vi "PIDAutoTune_OpenLoopStep.vi"(7 "Configuration Parameters":T2={"Controller Constant Type"=enum."Ziegler Nicols - Normal", "Type of Controller"=enum."PI", "CO Offset"=0.25, "Kn"=1.0, "Tuning Tolerance"=0.001, "Plant Tolerance"=0.001, "Newest Avg Time "=1, "Long Ave Time"=6}, 8 "Sampling Time dt (s)":dbl=0.02, 9 "Tune":bool, 10 "Measurement  (PV)":dbl, 11 "Control Output (Co)":dbl) -> (0 "Plant and Test Data":T4, 1 "New Tuning Parameters":T3, 2 "Tuning Done":bool, 3 "Adj CO":dbl, 4 "Error Occured":bool, 6 "Diagnostic":T1)   [LabVIEW 2019, in "Trajectory_Library.lvlib"]
uses:
  Trajectory_Library.lvlib
  <vilib>/addons/control/pid/NI_PID_autopid.lvlib
  <vilib>/ptbypt/NI_PtbyPt.lvlib
  <vilib>/Analysis/Matrix/NI_Matrix.lvlib
  <vilib>/addons/control/pid/autopid.llb/PID Autotuning Design (Auto).vi
  <vilib>/addons/control/pid/autopid.llb/PID Autotuning Design (Chien-Hrones-Reswick).vi
  <vilib>/Analysis/Matrix/Numeric/Conversions/Array To Matrix - RA.vi
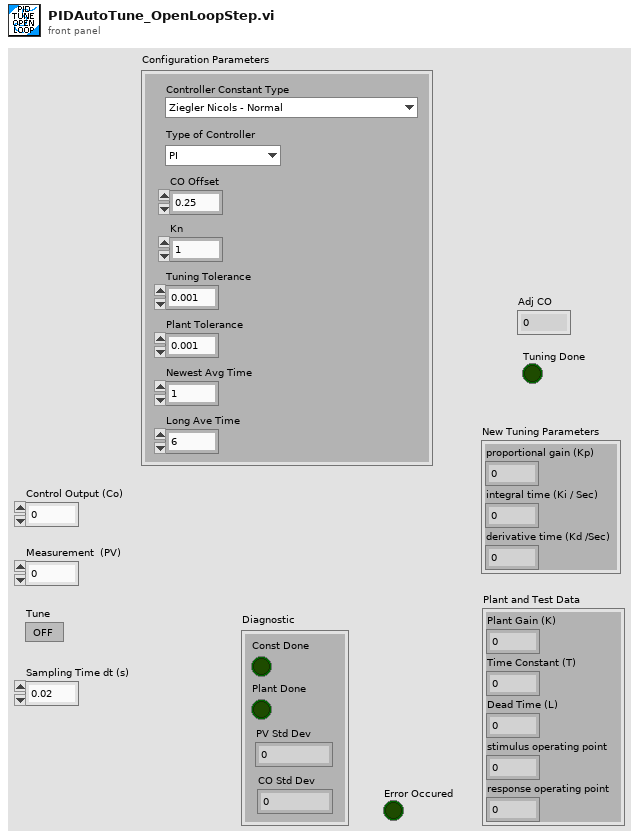
[diagram p1: front panel]
types:
  T1 = cluster{"Const Done":bool, "Plant Done":bool, "PV Std Dev":dbl, "CO Std Dev":dbl}
  T2 = cluster{"Controller Constant Type":enum16{"Ziegler Nicols - Fast", "Ziegler Nicols - Normal", "Ziegler Nicols - Slow", "CHR regulator - 0% overshoot", "CHR regulator - 20% overshoot", "CHR servo - 0 % overshoot", "CHR servo - 20% overshoot"}, "Type of Controller":enum16{"P", "PI", "PID"}, "CO Offset":dbl, "Kn":dbl, "Tuning Tolerance":dbl, "Plant Tolerance":dbl, "Newest Avg Time ":i32, "Long Ave Time":i32}
  T3 = cluster{"proportional gain (Kp)":dbl, "integral time (Ki / Sec)":dbl, "derivative time (Kd /Sec)":dbl}
  T4 = cluster{"Plant Gain (K)":dbl, "Time Constant (T)":dbl, "Dead Time (L)":dbl, "stimulus operating point":dbl, "response operating point":dbl}
  T5 = enum16{"Moving Average", "Low Pass 1st Order Butterworth", "Low Pass 2nd Order Butterworth", "High Pass 1st Order Butterworth", "High Pass 2nd Order Butterworth"}
  T6 = enum16{"Ziegler Nicols - Fast", "Ziegler Nicols - Normal", "Ziegler Nicols - Slow", "CHR regulator - 0% overshoot", "CHR regulator - 20% overshoot", "CHR servo - 0 % overshoot", "CHR servo - 20% overshoot"}
  T7 = cluster{"proportional gain (Kc)":dbl, "integral time (Ti, min)":dbl, "derivative time (Td, min)":dbl}
  T8 = cluster{"Plant Gain (K)":dbl, "Time Constant (T)":dbl, "Dead Time (L)":dbl}
  T9 = cluster{"Plant Gain (K)":dbl, "Time Constant (T)":dbl, "Dead Time (L)":dbl, "stimulus offset":dbl, "response offset":dbl}
  T10 = typedef "NI_Matrix.lvlib/RealMatrix.ctl" = dbl[][]
  T11 = cluster{"WithinTolerance":bool, "WithinTolerance":bool, "standard deviation":dbl, "standard deviation":dbl}
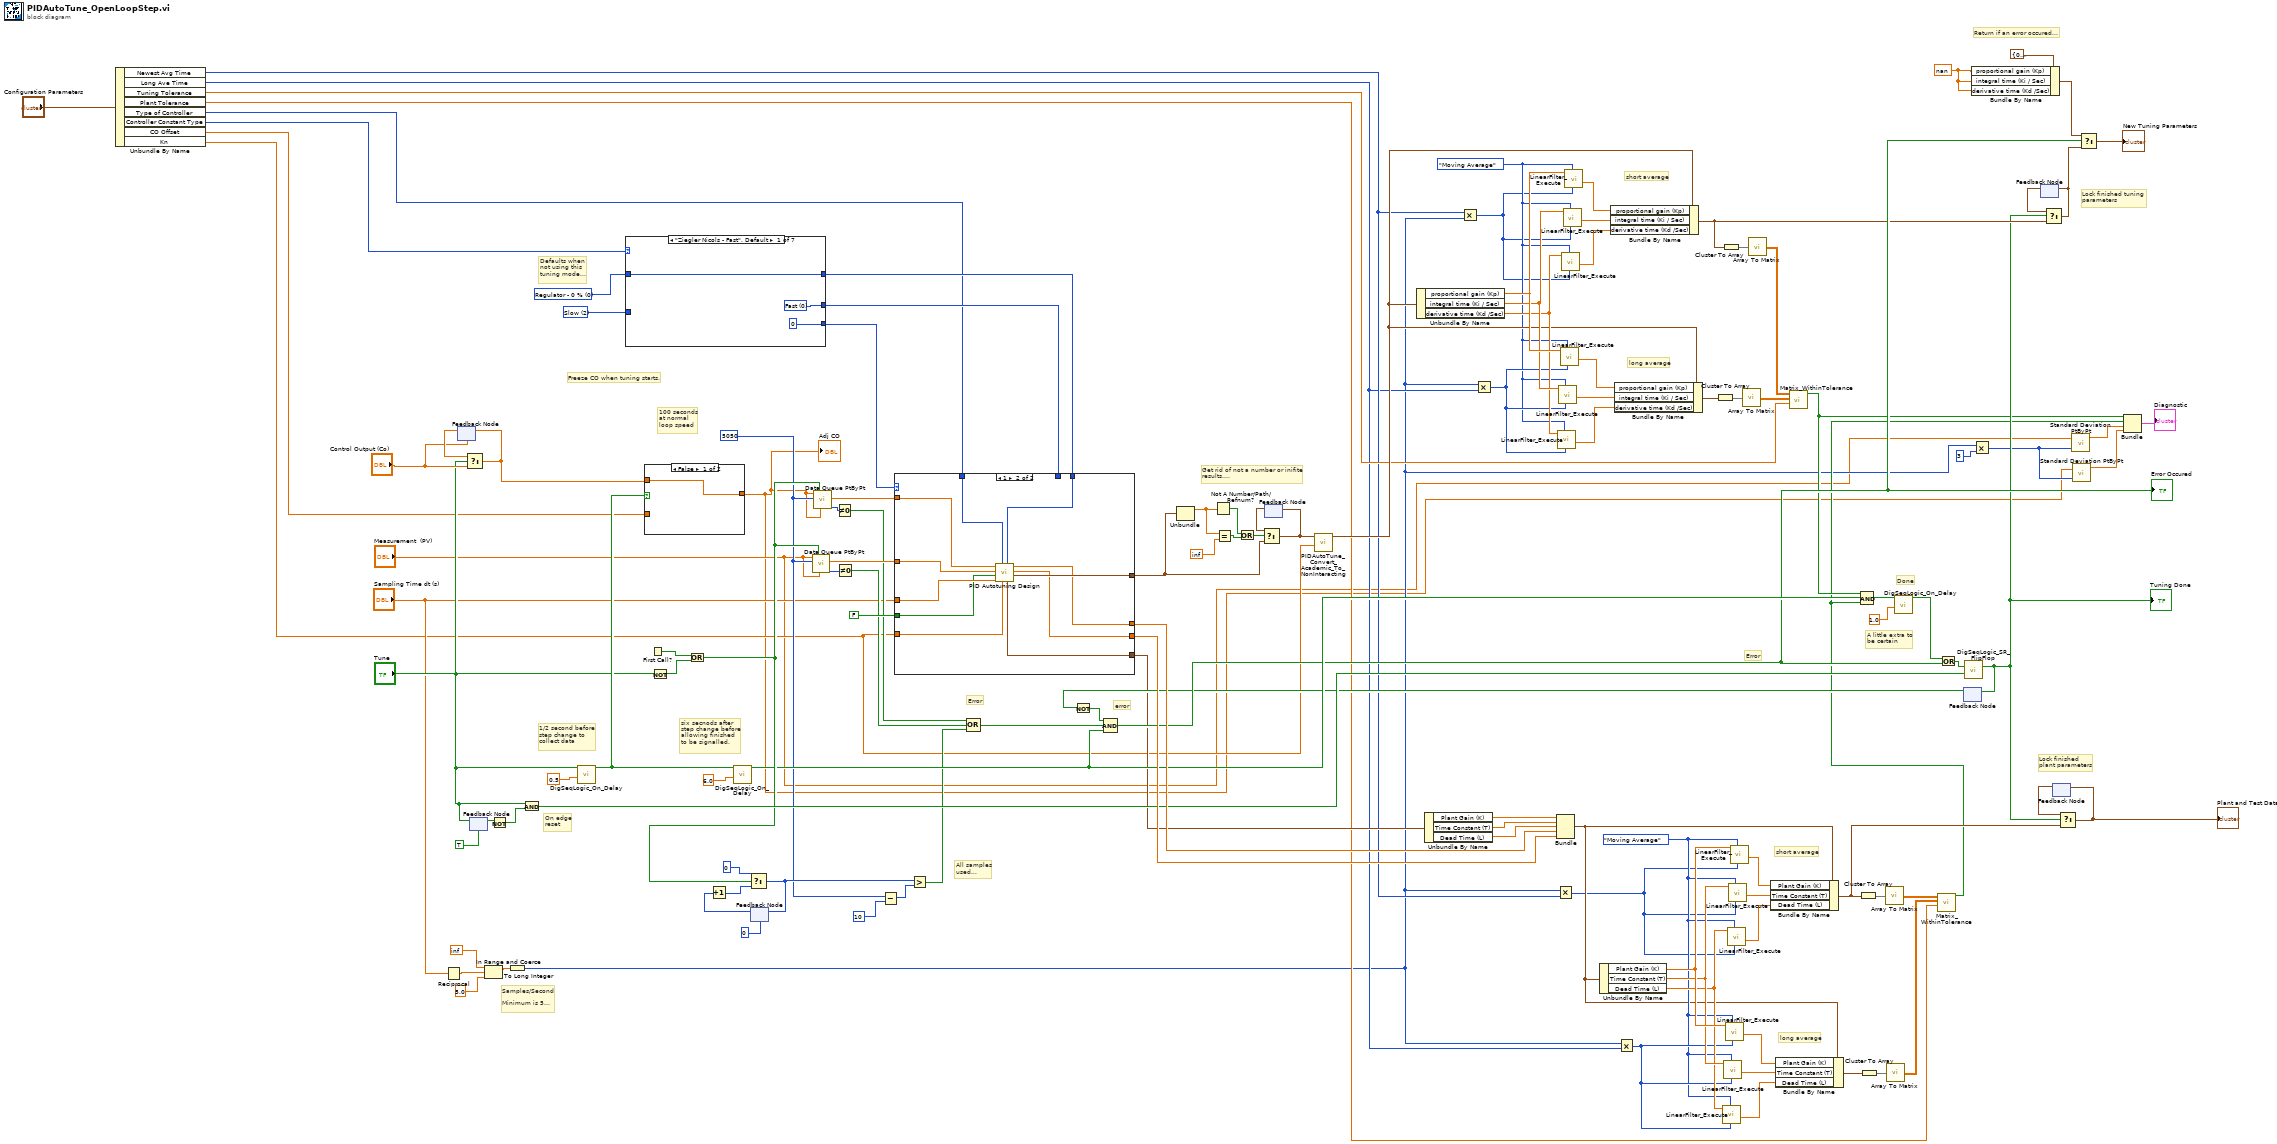
[diagram p0: block diagram]
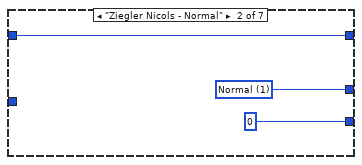
[diagram p2: hidden frame]
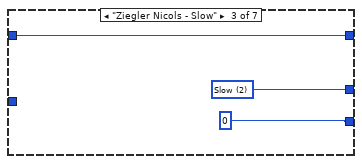
[diagram p3: hidden frame]
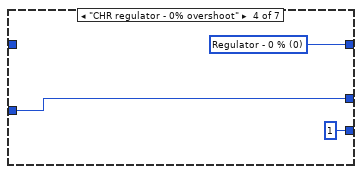
[diagram p4: hidden frame]
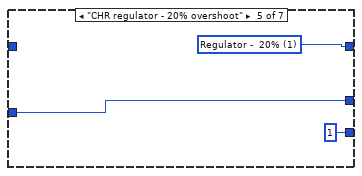
[diagram p5: hidden frame]
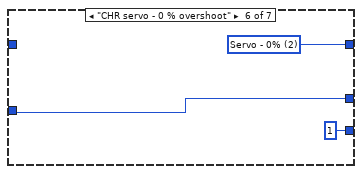
[diagram p6: hidden frame]
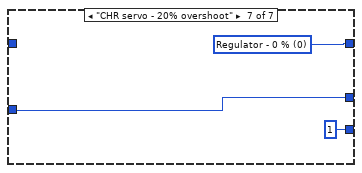
[diagram p7: hidden frame]
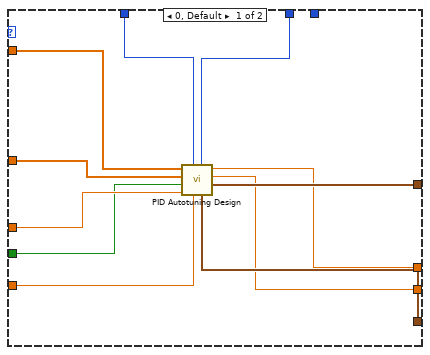
[diagram p8: hidden frame]
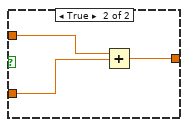
[diagram p9: hidden frame]
diagram:
  w31 = T5."Moving Average" ("Filter Type")
  w83 = nan
  w42 = T5."Moving Average" ("Filter Type")
  w98 = u16 2 items=["Fast", "Normal", "Slow"] ("Ziegler-Nichols Speed")
  w99 = u16 0 items=["Regulator - 0 %", "Regulator -  20%", "Servo - 0%", "Servo - 20%"] ("Tuning specifications")
  w70 = 5050 ("sample length")
  # "Get rid of not a number or inifite\nresults...."
  # "On edge\nreset"
  # "Error"
  # "All samples\nused..."
  # "Error"
  # "Done"
  # "Lock finished \nplant parameters"
  # "Lock finished tuning\nparameters"
  # "Samples/Second\n\nMinimum is 5..."
  # "long average"
  # "short average"
  # "long average"
  # "short average"
  # "error"
  # "Return if an error occured..."
  # "A little extra to\nbe certain"
  # "Defaults when\nnot using this\ntuning mode..."
  # "100 seconds\nat normal\nloop speed"
  # "Freeze CO when tuning starts."
  # "six secnods after\nstep change before\nallowing finished \nto be signalled."
  # "1/2 second before\nstep change to\ncollect data"
  n1 = Unbundle By Name("Configuration Parameters") -> ("Newest Avg Time"=w12:i32, "Long Ave Time"=w11:i32, "Tuning Tolerance"=w17:dbl, "Plant Tolerance"=w16:dbl, "Type of Controller"=w20:enum16{"P", "PI", "PID"}, "Controller Constant Type"=w21:T6, "CO Offset"=w19:dbl, "Kn"=w18:dbl)
  n2 = Reciprocal(x="Sampling Time dt (s)") -> (1/x=w60:dbl)
  n3 = feedback #1("Control Output (Co)") -> (w114:dbl)
  n4 = Select(t=w114, s="Tune", f="Control Output (Co)") -> (s? t:f=w115:dbl)
  n5 = feedback-in #1(w115) -> ()
  n6 = feedback-in #2("Tune") -> ()
  n7 = feedback #2(TRUE ("Tune")) -> (w111:bool)
  n8 = In Range and Coerce(upper limit=inf, x=w60, lower limit=5.0) -> (coerced(x)=w51:dbl)  [unwired: 1 out]
  n9 = Not(x=w111) -> (.not. x?=w109:bool)
  n10 = To Long Integer(number=w51) -> (32bit integer=w6:i32)
  n11 = And(x="Tune", y=w109) -> (x .and. y?=w108:bool)
  n12 = call "DigSeqLogic_On_Delay.vi"("Delay"=0.5, "Input"="Tune") -> ("Output"=w116:bool)  [unwired: 8 in, 1 out]
  n13 = case shown="\"Ziegler Nicols - Fast\", Default" w21 {
    tunnel: [w132 w135 w138 w139 w142 w145 w148] -> w102
    tunnel: [0 0 0 1 1 1 1] -> w101
    tunnel: [w130 w133 w136 w140 w143 w146 w149] -> w100
    tunnel: w99 -> [w130 w133 w136 _ _ _ _]
    tunnel: w98 -> [_ _ _ w139 w142 w145 w148]
    frame "Ziegler Nicols - Fast", Default {
      w132 = u16 0 items=["Fast", "Normal", "Slow"] ("Ziegler-Nichols Speed")
    }
    frame "Ziegler Nicols - Normal" {
      w135 = u16 1 items=["Fast", "Normal", "Slow"] ("Ziegler-Nichols Speed")
    }
    frame "Ziegler Nicols - Slow" {
      w138 = u16 2 items=["Fast", "Normal", "Slow"] ("Ziegler-Nichols Speed")
    }
    frame "CHR regulator - 0% overshoot" {
      w140 = u16 0 items=["Regulator - 0 %", "Regulator -  20%", "Servo - 0%", "Servo - 20%"] ("Tuning specifications")
    }
    frame "CHR regulator - 20% overshoot" {
      w143 = u16 1 items=["Regulator - 0 %", "Regulator -  20%", "Servo - 0%", "Servo - 20%"] ("Tuning specifications")
    }
    frame "CHR servo - 0 % overshoot" {
      w146 = u16 2 items=["Regulator - 0 %", "Regulator -  20%", "Servo - 0%", "Servo - 20%"] ("Tuning specifications")
    }
    frame "CHR servo - 20% overshoot" {
      w149 = u16 0 items=["Regulator - 0 %", "Regulator -  20%", "Servo - 0%", "Servo - 20%"] ("Tuning specifications")
    }
  }
  n14 = case shown="False" w116 {
    tunnel: w115 -> [w151 w154]
    tunnel: w19 -> [_ w153]
    tunnel: [w151 w152] -> w2
    frame False {
    }
    frame True {
      n15 = Add(x=w154, y=w153) -> (x+y=w152:dbl)
    }
  }
  "Adj CO" <- w2
  n16 = First Call?() -> (First Call?: T/F=w82:bool)
  n17 = Not(x="Tune") -> (.not. x?=w81:bool)
  n18 = Or(x=w82, y=w81) -> (x .or. y?=w79:bool)
  n19 = call "DigSeqLogic_On_Delay.vi"("Delay"=6.0, "Input"=w116) -> ("Output"=w77:bool)  [unwired: 8 in, 1 out]
  n20 = feedback #3(0) -> (w74:i32)
  n21 = Increment(x=w74) -> (x+1=w73:i32)
  n22 = Select(t=0, s=w79, f=w73) -> (s? t:f=w72:i32)
  n23 = feedback-in #3(w72) -> ()
  n24 = call <vilib>:"Data Queue PtByPt.vi"("initial queue element"="Measurement  (PV)", "initialize"=w79, "sample length"=w70, "input data point"="Measurement  (PV)") -> ("error"=w90:i32, "Current Queue"=w124:dbl[])  [unwired: 3 in, 3 out]
  n25 = call <vilib>:"Data Queue PtByPt.vi"("initial queue element"=w2, "initialize"=w79, "sample length"=w70, "input data point"=w2) -> ("error"=w91:i32, "Current Queue"=w125:dbl[])  [unwired: 3 in, 3 out]
  n26 = Not Equal To 0?(x=w91) -> (x != 0?=w67:bool)
  n27 = Not Equal To 0?(x=w90) -> (x != 0?=w66:bool)
  n28 = Subtract(x=w70, y=10) -> (x-y=w71:i32)
  n29 = case shown="1" w101 {
    tunnel: [w165 w176] -> w128
    tunnel: "Sampling Time dt (s)" -> [w164 w175]
    tunnel: w125 -> [w163 w174]
    tunnel: w124 -> [w162 w173]
    tunnel: w20 -> [w161 w172]
    tunnel: [w160 w171] -> w30
    tunnel: [w159 w170] -> w120
    tunnel: [w158 w169] -> w119
    tunnel: w18 -> [w157 w168]
    tunnel: w102 -> [w156 _]
    tunnel: w100 -> [_ w167]
    tunnel: FALSE ("closed-loop?") -> [w155 w166]
    frame 0, Default {
      n30 = call-poly <vilib>:"PID Autotuning Design.vi"("Ziegler-Nichols Speed"=w156, "Controller Gain (K)"=w157, "Type of Controller"=w161, "dt (s)"=w164, "closed-loop?"=w155, "Response signal"=w162, "Stimulus signal"=w163) -> ("PID gains"=w165:T7, "response operating point"=w158:dbl, "stimulus operating point"=w159:dbl, "Plant Parameters"=w160:T8)  [unwired: 1 in]
    }
    frame 1 {
      n31 = call-poly <vilib>:"PID Autotuning Design.vi"("Tuning specifications"=w167, "Controller Gain (K)"=w168, "Type of Controller"=w172, "dt (s)"=w175, "closed-loop?"=w166, "Response signal"=w173, "Stimulus signal"=w174) -> ("PID gains"=w176:T7, "response offset"=w169:dbl, "stimulus offset"=w170:dbl, "Plant Parameters"=w171:T8)  [unwired: 1 in]
    }
  }
  n32 = Greater?(x=w72, y=w71) -> (0:w68:bool)
  n33 = Compound Arithmetic op=OR(w67, w66, w68) -> (w78:bool)
  n34 = Unbundle(w128) -> ("proportional gain (Kc)"=w63:dbl)  [unwired: 2 out]
  n35 = Not A Number/Path/Refnum?(number/path/refnum=w63) -> (NaN/Path/Refnum?=w62:bool)
  n36 = Equal?(x=w63, y=inf) -> (x = y?=w92:bool)
  n37 = Or(x=w62, y=w92) -> (x .or. y?=w93:bool)
  n38 = feedback #4() -> (w127:T7)  [unwired: 1 in]
  n39 = Select(t=w127, s=w93, f=w128) -> (s? t:f=w129:T7)
  n40 = feedback-in #4(w129) -> ()
  n41 = call "PIDAutoTune_Convert_Academic_To_NonInteracting.vi"("Kn"=w18, "PID gains NI Academic"=w129) -> ("PID Gains Non Interacting"=w47:T3)  [unwired: 9 in]
  n42 = Unbundle By Name(w47) -> ("proportional gain (Kp)"=w54:dbl, "integral time (Ki / Sec)"=w53:dbl, "derivative time (Kd /Sec)"=w52:dbl)
  n43 = Unbundle By Name(w30) -> ("Plant Gain (K)"=w123:dbl, "Time Constant (T)"=w122:dbl, "Dead Time (L)"=w121:dbl)
  n44 = Multiply(x=w12, y=w6) -> (x*y=w15:i32)
  n45 = Multiply(x=w6, y=w11) -> (x*y=w50:i32)
  n46 = Bundle("Plant Gain (K)"=w123, "Time Constant (T)"=w122, "Dead Time (L)"=w121, "stimulus offset"=w120, "response offset"=w119) -> (w29:T9)  [unwired: 1 in]
  n47 = Multiply(x=w6, y=w12) -> (x*y=w13:i32)
  n48 = call "LinearFilter_Execute.vi"("Samples"=w50, "Filter Type"=w42, "Input"=w52) -> ("Output"=w55:dbl)  [unwired: 7 in, 1 out]
  n49 = call "LinearFilter_Execute.vi"("Samples"=w50, "Filter Type"=w42, "Input"=w53) -> ("Output"=w57:dbl)  [unwired: 7 in, 1 out]
  n50 = call "LinearFilter_Execute.vi"("Samples"=w50, "Filter Type"=w42, "Input"=w54) -> ("Output"=w56:dbl)  [unwired: 7 in, 1 out]
  n51 = call "LinearFilter_Execute.vi"("Samples"=w15, "Filter Type"=w42, "Input"=w52) -> ("Output"=w94:dbl)  [unwired: 7 in, 1 out]
  n52 = call "LinearFilter_Execute.vi"("Samples"=w15, "Filter Type"=w42, "Input"=w53) -> ("Output"=w95:dbl)  [unwired: 7 in, 1 out]
  n53 = call "LinearFilter_Execute.vi"("Samples"=w15, "Filter Type"=w42, "Input"=w54) -> ("Output"=w96:dbl)  [unwired: 7 in, 1 out]
  n54 = Unbundle By Name(w29) -> ("Plant Gain (K)"=w35:dbl, "Time Constant (T)"=w34:dbl, "Dead Time (L)"=w33:dbl)
  n55 = Bundle By Name(cluster=w47, "proportional gain (Kp)"=w96, "integral time (Ki / Sec)"=w95, "derivative time (Kd /Sec)"=w94) -> (w46:T3)
  n56 = Bundle By Name(cluster=w47, "proportional gain (Kp)"=w56, "integral time (Ki / Sec)"=w57, "derivative time (Kd /Sec)"=w55) -> (w49:T3)
  n57 = Multiply(x=w6, y=w11) -> (x*y=w32:i32)
  n58 = Cluster To Array(cluster=w49) -> (array=w48:dbl[])
  n59 = Cluster To Array(cluster=w46) -> (array=w45:dbl[])
  n60 = call "LinearFilter_Execute.vi"("Samples"=w32, "Filter Type"=w31, "Input"=w33) -> ("Output"=w36:dbl)  [unwired: 7 in, 1 out]
  n61 = call "LinearFilter_Execute.vi"("Samples"=w32, "Filter Type"=w31, "Input"=w34) -> ("Output"=w38:dbl)  [unwired: 7 in, 1 out]
  n62 = call "LinearFilter_Execute.vi"("Samples"=w32, "Filter Type"=w31, "Input"=w35) -> ("Output"=w37:dbl)  [unwired: 7 in, 1 out]
  n63 = call "LinearFilter_Execute.vi"("Samples"=w13, "Filter Type"=w31, "Input"=w33) -> ("Output"=w39:dbl)  [unwired: 7 in, 1 out]
  n64 = call "LinearFilter_Execute.vi"("Samples"=w13, "Filter Type"=w31, "Input"=w34) -> ("Output"=w40:dbl)  [unwired: 7 in, 1 out]
  n65 = call "LinearFilter_Execute.vi"("Samples"=w13, "Filter Type"=w31, "Input"=w35) -> ("Output"=w41:dbl)  [unwired: 7 in, 1 out]
  n66 = call-poly <vilib>:"Array To Matrix.vi"("Real 1D Array"=w48) -> ("Real Matrix (Column Vector)"=w44:T10)
  n67 = call-poly <vilib>:"Array To Matrix.vi"("Real 1D Array"=w45) -> ("Real Matrix (Column Vector)"=w43:T10)
  n68 = Bundle By Name(cluster=w29, "Plant Gain (K)"=w41, "Time Constant (T)"=w40, "Dead Time (L)"=w39) -> (w25:T9)
  n69 = Bundle By Name(cluster=w29, "Plant Gain (K)"=w37, "Time Constant (T)"=w38, "Dead Time (L)"=w36) -> (w26:T9)
  n70 = call "Matrix_WithinTolerance.vi"("Tolerance"=w17, "Matrix B"=w44, "Matrix A"=w43) -> ("WithinTolerance"=w9:bool)  [unwired: 7 in, 1 out]
  n71 = Cluster To Array(cluster=w25) -> (array=w28:dbl[])
  n72 = Cluster To Array(cluster=w26) -> (array=w27:dbl[])
  n73 = call-poly <vilib>:"Array To Matrix.vi"("Real 1D Array"=w28) -> ("Real Matrix (Column Vector)"=w24:T10)
  n74 = call-poly <vilib>:"Array To Matrix.vi"("Real 1D Array"=w27) -> ("Real Matrix (Column Vector)"=w23:T10)
  n75 = call "Matrix_WithinTolerance.vi"("Tolerance"=w16, "Matrix B"=w23, "Matrix A"=w24) -> ("WithinTolerance"=w8:bool)  [unwired: 7 in, 1 out]
  n76 = Compound Arithmetic op=AND(w9, w77, w8) -> (w104:bool)
  n77 = call "DigSeqLogic_On_Delay.vi"("Delay"=1.0, "Input"=w104) -> ("Output"=w88:bool)  [unwired: 8 in, 1 out]
  n78 = feedback #5() -> (w64:bool)  [unwired: 1 in]
  n79 = Not(x=w64) -> (.not. x?=w65:bool)
  n80 = Compound Arithmetic op=AND(w65, w78, w77) -> (w76:bool)
  "Error Occured" <- w76
  n81 = Or(x=w88, y=w76) -> (x .or. y?=w89:bool)
  n82 = call "DigSeqLogic_SR_FlipFlop.vi"("Set"=w89, "Reset"=w108) -> ("Output"=w14:bool)  [unwired: 12 in, 1 out]
  "Tuning Done" <- w14
  n83 = feedback-in #5(w14) -> ()
  n84 = Bundle By Name(cluster=T3 {"proportional gain (Kp)"=0.0, "integral time (Ki / Sec)"=0.0, "derivative time (Kd /Sec)"=0.0} ("t"), "proportional gain (Kp)"=w83, "integral time (Ki / Sec)"=w83, "derivative time (Kd /Sec)"=w83) -> (w84:T3)
  n85 = Multiply(x=w6, y=3) -> (x*y=w3:i32)
  n86 = feedback #6() -> (w105:T3)  [unwired: 1 in]
  n87 = Select(t=w105, s=w14, f=w46) -> (s? t:f=w86:T3)
  n88 = feedback-in #6(w86) -> ()
  n89 = feedback #7() -> (w106:T9)  [unwired: 1 in]
  n90 = Select(t=w106, s=w14, f=w25) -> (s? t:f=w107:T9)
  "Plant and Test Data" <- w107
  n91 = feedback-in #7(w107) -> ()
  n92 = call <vilib>:"Standard Deviation PtByPt.vi"("x"="Measurement  (PV)", "sample length"=w3) -> ("standard deviation"=w7:dbl)  [unwired: 1 in, 2 out]
  n93 = call <vilib>:"Standard Deviation PtByPt.vi"("x"=w2, "sample length"=w3) -> ("standard deviation"=w1:dbl)  [unwired: 1 in, 2 out]
  n94 = Select(t=w84, s=w76, f=w86) -> (s? t:f=→"New Tuning Parameters":T3)
  n95 = Bundle("WithinTolerance"=w9, "WithinTolerance"=w8, "standard deviation"=w7, "standard deviation"=w1) -> (→"Diagnostic":T11)  [unwired: 1 in]
